vi "parse argument.vi"(11 "Arguments":string[](array[string])) -> (2 "values":string[](array[string]), 3 "flags":string[](array[string]))   [LabVIEW 2013]
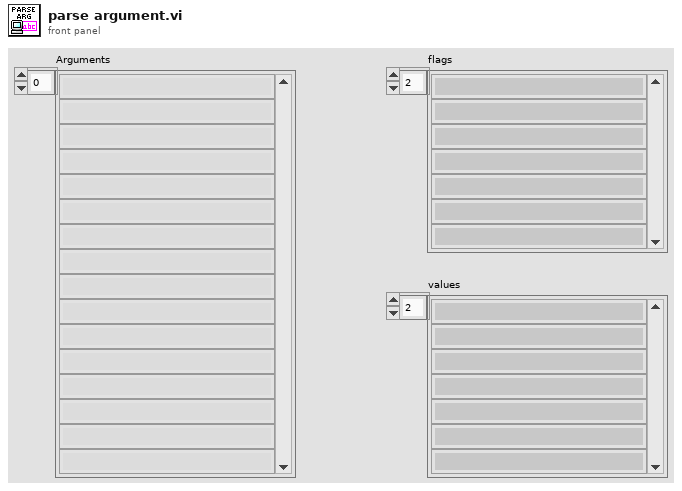
[diagram p1: front panel]
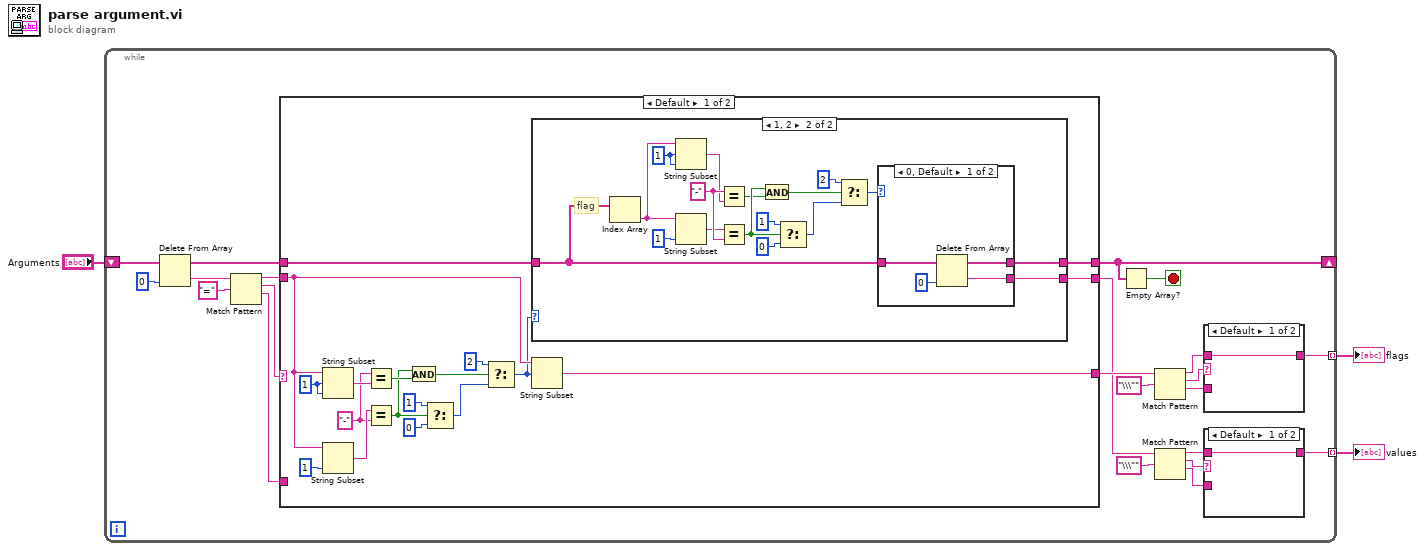
[diagram p0: block diagram]
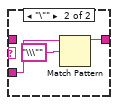
[diagram p2: hidden frame]
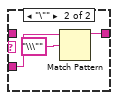
[diagram p3: hidden frame]
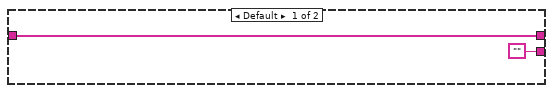
[diagram p4: hidden frame]
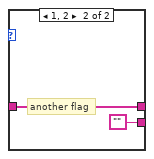
[diagram p5: hidden frame]
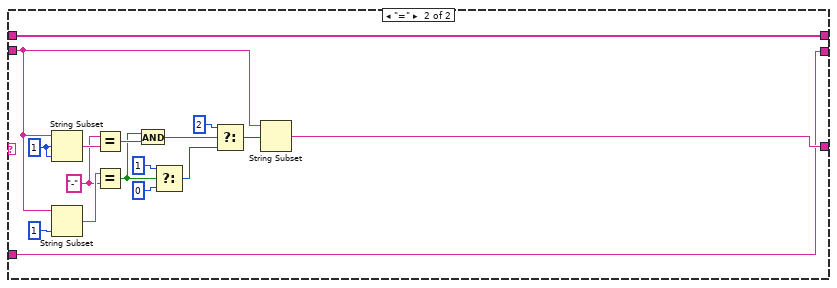
[diagram p6: hidden frame]
diagram:
  n1 = while {
    shift-right: [w5] -> _
    shift-left: "Arguments" -> [w25]
    tunnel: [w6] -> w2 mode=indexing
    tunnel: [w8] -> w1 mode=indexing
    stop <- w4 stop-if-true
    n2 = Delete From Array(array=w25, index=0) -> (deleted portion=w23:string, array with subset deleted=w20:string[])  [unwired: 1 in]
    n3 = Match Pattern(string=w23, regular expression="=") -> (before substring=w19:string, match substring=w21:string, after substring=w18:string)  [unwired: 1 in, 1 out]
    n4 = case shown="Default" w21 {
      tunnel: w20 -> [w36 w93]
      tunnel: [w35 w93] -> w5
      tunnel: w19 -> [w39 w79]
      tunnel: w18 -> [_ w77]
      tunnel: [w37 w77] -> w7
      tunnel: [w34 w78] -> w9
      frame Default {
        w47 = "-" ("y")
        w49 = 1 ("length (rest)")
        n5 = String Subset(string=w39, offset (0)=w49, length (rest)=w49) -> (substring=w48:string)
        n6 = String Subset(string=w39, length (rest)=1 ("length (rest)")) -> (substring=w50:string)  [unwired: 1 in]
        n7 = Equal?(x=w47, y=w48) -> (x = y?=w44:bool)
        n8 = Equal?(x=w50, y=w47) -> (x = y?=w43:bool)
        n9 = And(x=w43, y=w44) -> (x .and. y?=w42:bool)
        n10 = Select(t=1 ("length (rest)"), s=w43, f=0 ("length (rest)")) -> (s? t:f=w41:i32)
        n11 = Select(t=2, s=w42, f=w41) -> (s? t:f=w38:i32)
        n12 = case shown="1, 2" w38 {
          tunnel: ["" w54] -> w37
          tunnel: w36 -> [w52 w55]
          tunnel: [w52 w56] -> w35
          frame Default {
          }
          frame 1, 2 {
            w63 = "-" ("y")
            w61 = 1 ("length (rest)")
            # "flag"
            n13 = Index Array(array=w55) -> (element=w58:string)  [unwired: 1 in]
            n14 = String Subset(string=w58, offset (0)=w61, length (rest)=w61) -> (substring=w62:string)
            n15 = String Subset(string=w58, length (rest)=1 ("length (rest)")) -> (substring=w60:string)  [unwired: 1 in]
            n16 = Equal?(x=w63, y=w62) -> (x = y?=w66:bool)
            n17 = Equal?(x=w60, y=w63) -> (x = y?=w67:bool)
            n18 = And(x=w67, y=w66) -> (x .and. y?=w68:bool)
            n19 = Select(t=1 ("length (rest)"), s=w67, f=0 ("length (rest)")) -> (s? t:f=w69:i32)
            n20 = Select(t=2, s=w68, f=w69) -> (s? t:f=w57:i32)
            n21 = case shown="0, Default" w57 {
              tunnel: [w73 w76] -> w56
              tunnel: w55 -> [w74 w76]
              tunnel: [w72 ""] -> w54
              frame 0, Default {
                n22 = Delete From Array(array=w74, index=0) -> (deleted portion=w72:string, array with subset deleted=w73:string[])  [unwired: 1 in]
              }
              frame 1, 2 {
                # "another flag"
              }
            }
          }
        }
        n23 = String Subset(string=w39, offset (0)=w38) -> (substring=w34:string)  [unwired: 1 in]
      }
      frame "=" {
        w88 = "-" ("y")
        w90 = 1 ("length (rest)")
        n24 = String Subset(string=w79, offset (0)=w90, length (rest)=w90) -> (substring=w89:string)
        n25 = String Subset(string=w79, length (rest)=1 ("length (rest)")) -> (substring=w91:string)  [unwired: 1 in]
        n26 = Equal?(x=w88, y=w89) -> (x = y?=w85:bool)
        n27 = Equal?(x=w91, y=w88) -> (x = y?=w84:bool)
        n28 = And(x=w84, y=w85) -> (x .and. y?=w83:bool)
        n29 = Select(t=1 ("length (rest)"), s=w84, f=0 ("length (rest)")) -> (s? t:f=w82:i32)
        n30 = Select(t=2, s=w83, f=w82) -> (s? t:f=w80:i32)
        n31 = String Subset(string=w79, offset (0)=w80) -> (substring=w78:string)  [unwired: 1 in]
      }
    }
    n32 = Empty Array?(array=w5) -> (empty?=w4:bool)
    n33 = Match Pattern(string=w9, regular expression="\\\"") -> (before substring=w11:string, match substring=w12:string, after substring=w10:string)  [unwired: 1 in, 1 out]
    n34 = Match Pattern(string=w7, regular expression="\\\"") -> (before substring=w16:string, match substring=w15:string, after substring=w17:string)  [unwired: 1 in, 1 out]
    n35 = case shown="Default" w12 {
      tunnel: [w26 w27] -> w8
      tunnel: w11 -> [w26 _]
      tunnel: w10 -> [_ w28]
      frame Default {
      }
      frame "\"" {
        n36 = Match Pattern(string=w28, regular expression="\\\"") -> (before substring=w27:string)  [unwired: 1 in, 3 out]
      }
    }
    n37 = case shown="Default" w15 {
      tunnel: [w30 w31] -> w6
      tunnel: w16 -> [w30 _]
      tunnel: w17 -> [_ w32]
      frame Default {
      }
      frame "\"" {
        n38 = Match Pattern(string=w32, regular expression="\\\"") -> (before substring=w31:string)  [unwired: 1 in, 3 out]
      }
    }
  }
  "flags" <- w1
  "values" <- w2
